vi "Log.vi"(8 "error in (no error)":errorcluster, 10 "Log Text":string, 11 "Rotating File Sink in":refnum<class "Rotating Daily File Sink.lvclass">) -> (0 "error out":errorcluster, 3 "Rotating File Sink out":refnum<class "Rotating Daily File Sink.lvclass">)   [LabVIEW 2020, in "LV Log.lvlib" / "Rotating Daily File Sink.lvclass"]
uses:
  Rotating Daily File Sink.lvclass
  File Sink/File Sink.lvclass
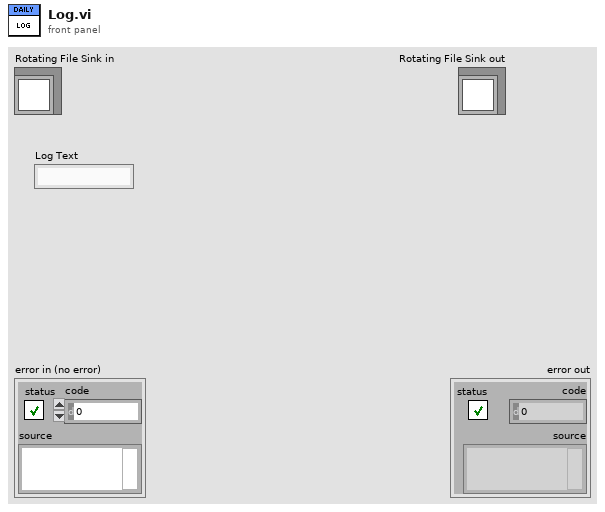
[diagram p1: front panel]
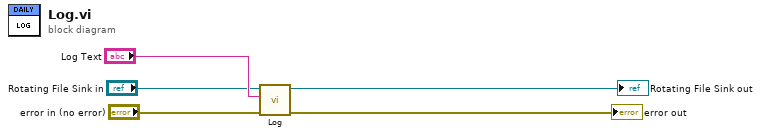
[diagram p0: block diagram]
diagram:
  n1 = call-parent "Log.vi"("error in (no error)"="error in (no error)", "Log Text"="Log Text", "File Sink in"="Rotating File Sink in") -> ("error out"=→"error out":errorcluster, "File Sink out"=→"Rotating File Sink out":refnum<class "Rotating Daily File Sink.lvclass">)  [unwired: 7 in]
